vi "checkFinishNormalDefensivePlay.vi"(8 "error in (no error)":errorcluster, 10 "Game":refnum<class "Game.lvclass">, 11 "NormalDefensivePlay in":refnum<class "NormalDefensivePlay.lvclass">) -> (0 "error out":errorcluster, 2 "Boolean":bool, 3 "NormalDefensivePlay out":refnum<class "NormalDefensivePlay.lvclass">)   [LabVIEW 2018, in "NormalDefensivePlay.lvclass"]
uses:
  NormalDefensivePlay.lvclass
  Game_class/Game.lvclass
  NormalDefensiveWithDuelistPlay_class/NormalDefensiveWithDuelistPlay.lvclass
  Referee_class/command_interpreted.ctl
  Game_class/Game.lvclass/Game.ctl
  Referee_class/Referee.lvclass/Referee.ctl
  Events_class/Events.lvclass/Events.ctl
  Game_class/Read Referee.vi
  Game_class/Read EventsRef.vi
  Events_class/Read ball_out.vi
  Referee_class/Read command_interpreted.vi
  Referee_class/Referee.lvclass
  Events_class/Events.lvclass
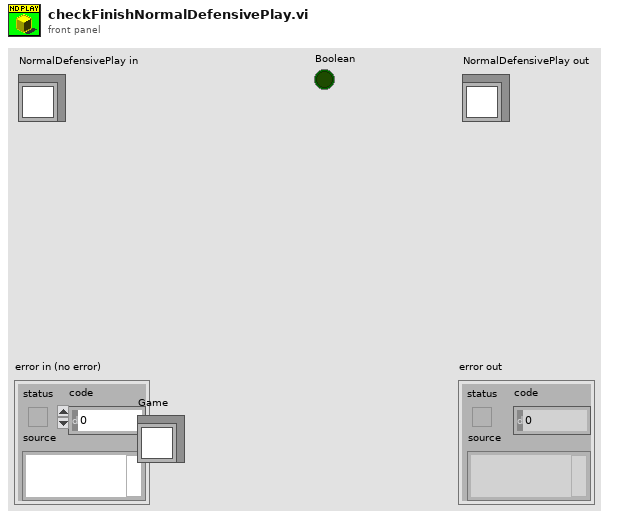
[diagram p1: front panel]
types:
  T1 = typedef "command_interpreted.ctl" = enum16{"Goal Ally", "Goal Enemy", "Ball Placement Enemy", "Ball Placement Ally", "Normal Half Time", "Extra Time  Break", "Extra Half Time", "None", "Post Game", "PKA Normal Start", "Prepare Kickoff Ally", "PKE Normal Start", "Prepare Kickoff Enemy", "Force Start", "Halt", "Timeout", "Prepare Penalty Ally", "Prepare Penalty Enemy", "PPA NormalStart", "PPE Normal Start", "Indirect Free Ally", "Direct Free Enemy", "Direct Free Ally", "Indirect Free Enemy", "Stop"}
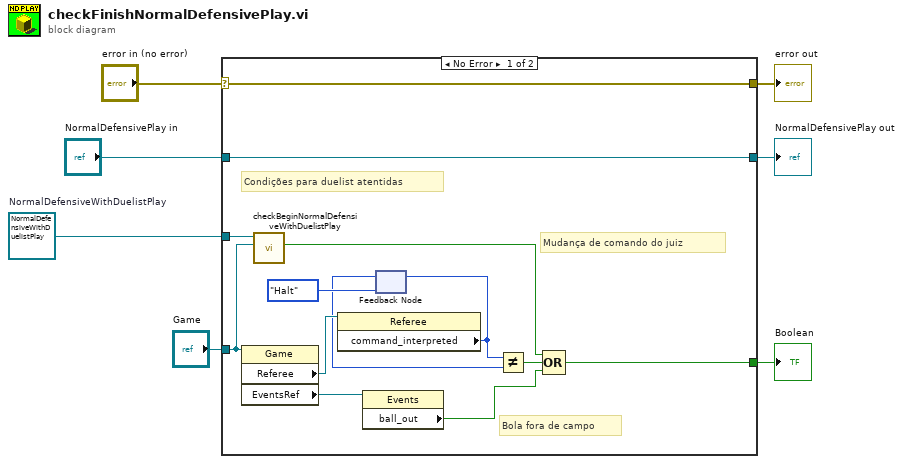
[diagram p0: block diagram]
diagram:
  w1 = refnum<class "NormalDefensiveWithDuelistPlay.lvclass"> refnum  # NormalDefensiveWithDuelistPlay
  n1 = case shown="No Error" "error in (no error)" {
    selector: "error in (no error)" -> [w19 w22]
    tunnel: [w19 w22] -> w6
    tunnel: [w20 w21] -> w4
    tunnel: "NormalDefensivePlay in" -> [w20 w21]
    tunnel: "Game" -> [w9 _]
    tunnel: [w11 _] -> w2
    tunnel: w1 -> [w10 _]
    frame No Error {
      # "Condições para duelist atentidas"
      # "Bola fora de campo"
      # "Mudança de comando do juiz"
      n2 = property class="Game"(reference=w9) -> ("Referee"=w18:refnum<class "Referee.lvclass">, "EventsRef"=w14:refnum<class "Events.lvclass">)  [unwired: 1 in, 2 out]
      n3 = call "checkBeginNormalDefensiveWithDuelistPlay.vi"("Game"=w9, "NormalDefensiveWithDuelistPlay in"=w10) -> ("Boolean"=w8:bool)  [unwired: 7 in, 2 out]
      n4 = property class="Referee"(reference=w18) -> ("command_interpreted"=w17:T1)  [unwired: 1 in, 2 out]
      n5 = property class="Events"(reference=w14) -> ("ball_out"=w13:bool)  [unwired: 1 in, 2 out]
      n6 = feedback #1(command_interpreted."Halt" ("command_interpreted")) -> (w12:T1)
      n7 = feedback-in #1(w17) -> ()
      n8 = Not Equal?(x=w17, y=w12) -> (x != y?=w15:bool)
      n9 = Compound Arithmetic op=OR(w8, w15, w13) -> (w11:bool)
    }
    frame Error {
    }
  }
  "error out" <- w6
  "NormalDefensivePlay out" <- w4
  "Boolean" <- w2
